vi "VI-Add XControl Event.vi"(0 "XCtl Path":path=path "C:/Users/Ken/Desktop/New XControl/New XControl.xctl", 7 "Name":string, 11 "error in (no error)":errorcluster) -> (15 "error out":errorcluster)   [LabVIEW 2015]
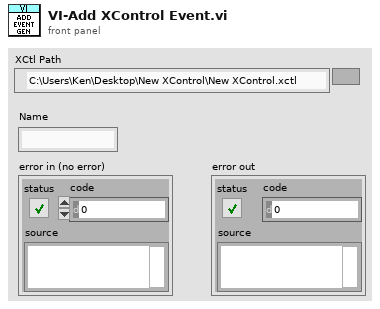
[diagram p1: front panel]
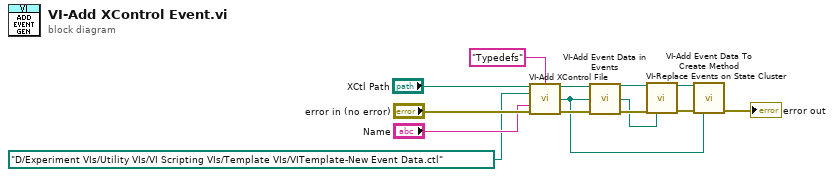
[diagram p0: block diagram]
diagram:
  n1 = call "VI-Add XControl File.vi"("XCtl Path in"="XCtl Path", "Add to folder"="Typedefs", "Template"=path "D:/Experiment VIs/Utility VIs/VI Scripting VIs/Template VIs/VITemplate-New Event Data.ctl" ("Typedef Path"), "Name"="Name", "error in (no error)"="error in (no error)") -> ("XCtl Path out"=w8:path, "local path"=w2:path, "error out"=w7:errorcluster)  [unwired: 8 in]
  n2 = call "VI-Add Event Data in Events.vi"("XCtl Path in"=w8, "Event Data typedef"=w2, "error in (no error)"=w7) -> ("XCtl Path out"=w13:path, "Events typedef"=w9:path, "error out"=w14:errorcluster)  [unwired: 10 in]
  n3 = call "VI-Replace Events on State Cluster.vi"("XCtl Path in"=w13, "error in (no error)"=w14, "Event Data typedef"=w9) -> ("XCtl Path out"=w11:path, "error out"=w12:errorcluster)  [unwired: 11 in]
  n4 = call "VI-Add Event Data To Create Method.vi"("XCtl Path in"=w11, "error in (no error)"=w12, "Event Data typedef"=w2) -> ("error out"=→"error out":errorcluster)  [unwired: 11 in, 1 out]
